vi "Build Tree.vi"(8 "error in (no error)":errorcluster, 10 "Tree Reference":refnum<vi>, 11 "Base Tree in":refnum<class "Base Tree.lvclass">) -> (0 "error out":errorcluster, 3 "Base Tree out":refnum<class "Base Tree.lvclass">)   [LabVIEW 2017, in "opcua.lvlib" / "Browser Core.lvlib" / "Base Tree.lvclass"]
doc: "Write Tree hierarchy to input control reference. The Tree's root node will be used as the top level item."
uses:
  Base Tree.lvclass
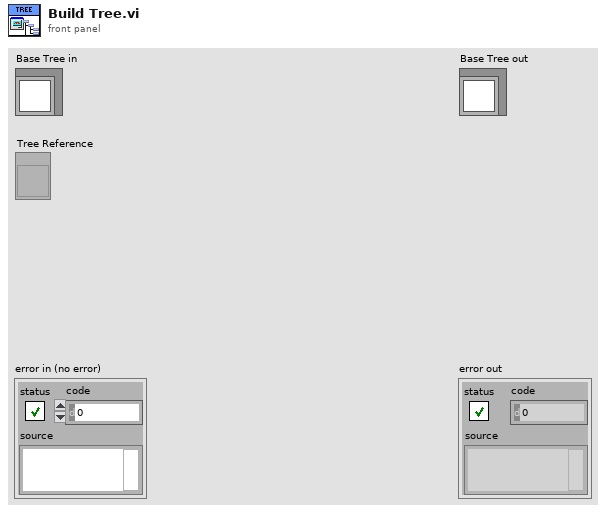
[diagram p1: front panel]
types:
  T1 = cluster{"Left Cell String":string, "Child Text":string[], "Child Tag":string, "Item Indent":i32, "Child Only?":bool, "Glyph Index":i32}[]
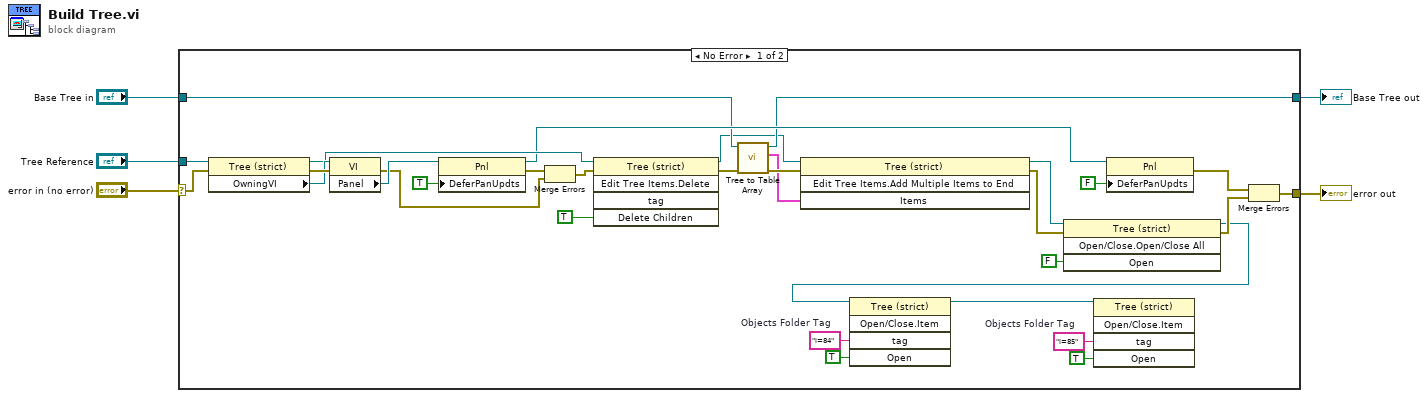
[diagram p0: block diagram]
diagram:
  n1 = case shown="No Error" "error in (no error)" {
    selector: "error in (no error)" -> [w24 w38]
    tunnel: [w22 w38] -> w4
    tunnel: [w18 w37] -> w2
    tunnel: "Base Tree in" -> [w19 w37]
    tunnel: "Tree Reference" -> [w29 _]
    frame No Error {
      w8 = "i=84"  # Objects Folder Tag
      w11 = "i=85"  # Objects Folder Tag
      n2 = property class="Tree (strict)"(reference=w29, error in=w24) -> (reference out=w28:refnum<vi>, error out=w36:errorcluster, "OwningVI"=w35:refnum<vi>)
      n3 = property class="VI"(reference=w35, error in=w36) -> (error out=w25:errorcluster, "Panel"=w32:refnum<vi>)  [unwired: 1 out]
      n4 = property class="Pnl"(reference=w32, "DeferPanUpdts"=TRUE ("Defer Panel Updates")) -> (reference out=w27:refnum<vi>, error out=w31:errorcluster)  [unwired: 1 in]
      n5 = Merge Errors(w31, w25) -> (w26:errorcluster)
      n6 = invoke class="Tree (strict)" method="Edit Tree Items.Delete"(reference=w28, error in=w26, "Delete Children"=TRUE ("Delete Children?")) -> (reference out=w16:refnum<vi>, error out=w21:errorcluster)  [unwired: 2 in, 3 out]
      n7 = call-dynamic "Tree to Table Array.vi"("error in (no error)"=w21, "Base Tree in"=w19) -> ("error out"=w20:errorcluster, "Tree Items"=w17:T1, "Base Tree out"=w18:refnum<class "Base Tree.lvclass">)  [unwired: 7 in]
      n8 = invoke class="Tree (strict)" method="Edit Tree Items.Add Multiple Items to End"(reference=w16, error in=w20, "Items"=w17) -> (reference out=w15:refnum<vi>, error out=w13:errorcluster)  [unwired: 1 in, 2 out]
      n9 = invoke class="Tree (strict)" method="Open/Close.Open/Close All"(reference=w15, error in=w13, "Open"=FALSE ("Open?")) -> (reference out=w7:refnum<vi>, error out=w12:errorcluster)  [unwired: 1 in, 2 out]
      n10 = invoke class="Tree (strict)" method="Open/Close.Item"(reference=w7, "tag"=w8, "Open"=TRUE ("Open?")) -> (reference out=w6:refnum<vi>)  [unwired: 2 in, 4 out]
      n11 = invoke class="Tree (strict)" method="Open/Close.Item"(reference=w6, "tag"=w11, "Open"=TRUE ("Open?")) -> ()  [unwired: 2 in, 5 out]
      n12 = property class="Pnl"(reference=w27, "DeferPanUpdts"=FALSE ("Defer Panel Updates")) -> (error out=w23:errorcluster)  [unwired: 1 in, 1 out]
      n13 = Merge Errors(w23, w12) -> (w22:errorcluster)
    }
    frame Error {
      # "Do Not Edit Tree on Error In"
    }
  }
  "error out" <- w4
  "Base Tree out" <- w2
